vi "Send Time-Delayed Response.vi"(7 "Message Priority (Normal)":T1=enum."Normal", 8 "error in (no error)":errorcluster, 10 "Milliseconds To Wait":i32=1000, 11 "Message Enqueuer":refnum<class "Message Enqueuer.lvclass">) -> (0 "error out":errorcluster, 3 "Message Enqueuer out":refnum<class "Message Enqueuer.lvclass">)   [LabVIEW 2015, in "Time-Delayed Response Msg.lvclass"]
doc: "This VI sends the message to an actor."
uses:
  Time-Delayed Response Msg.lvclass
  <vilib>/ActorFramework/Message Enqueuer/Message Enqueuer.lvclass
  <vilib>/ActorFramework/Message Enqueuer/Message Priority.ctl
  <vilib>/ActorFramework/Time-Delayed Send Message/Time-Delay Override Options.ctl
panel:
  out "Delivery Notifier":refnum<notifier>
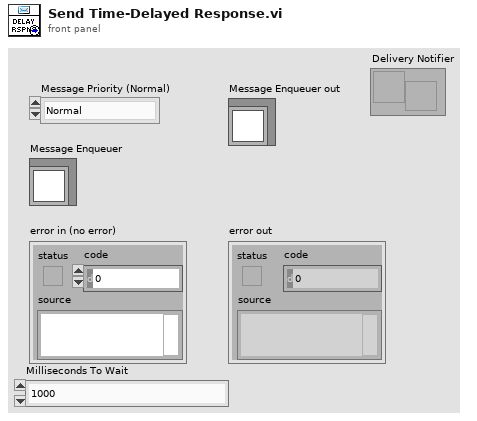
[diagram p1: front panel]
types:
  T1 = typedef "Actor Framework.lvlib/Message Enqueuer.lvclass/Message Priority.ctl" = enum16{"Low", "Normal", "High"}
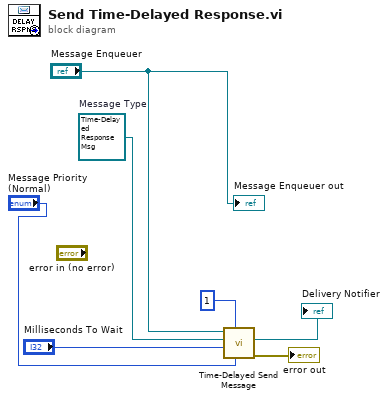
[diagram p0: block diagram]
diagram:
  w2 = refnum<class "Time-Delayed Response Msg.lvclass"> refnum  # Message Type
  n1 = call <vilib>:"Time-Delayed Send Message.vi"("Message Priority (Normal)"="Message Priority (Normal)", "# Copies (0 = infinite repeat)"=u32 1, "Milliseconds To Wait"="Milliseconds To Wait", "Message"=w2, "Message Enqueuer"="Message Enqueuer") -> ("error out"=→"error out":errorcluster, "Delivery Notifier"=→"Delivery Notifier":refnum<notifier>)  [unwired: 5 in]
  "Message Enqueuer out" <- "Message Enqueuer"
